vi "Agilent SNA Read Learn String.vi"(6 "Get SWP Learn String? (T)":bool=TRUE, 7 "Agilent SNA & SWP":T2, 8 "error in (no error)":errorcluster, 11 "VISA Resource Names":T1) -> (0 "error out":errorcluster, 1 "SWP Learn String":string, 2 "SNA Learn String":string, 3 "dup VISA Resource Names":T1)   [LabVIEW 2011]
uses:
  TypeDefs/Agilent SNA Instrument Info.ctl
  TypeDefs/Agilent SNA VISA.ctl
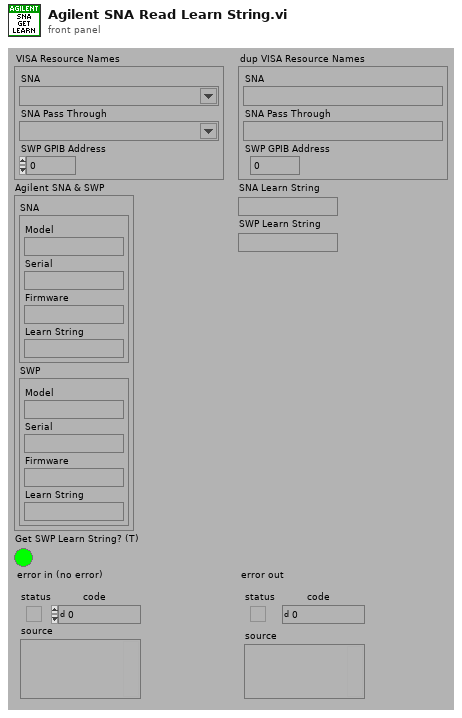
[diagram p1: front panel]
types:
  T1 = typedef "Agilent SNA VISA.ctl" = cluster{"SNA":refnum<visa-resource-name>, "SNA Pass Through":refnum<visa-resource-name>, "SWP GPIB Address":i32}
  T2 = typedef "Agilent SNA Instrument Info.ctl" = cluster{"SNA":cluster{"Model":string, "Serial":string, "Firmware":string, "Learn String":string}, "SWP":cluster{"Model":string, "Serial":string, "Firmware":string, "Learn String":string}}
  T3 = typedef "Agilent SNA Model.ctl" = enum16{"Not Supported", "8757X"}
  T4 = typedef "Agilent SNA SWP Model.ctl" = enum16{"Not Supported", "836XXX", "8375XX", "E82X7D"}
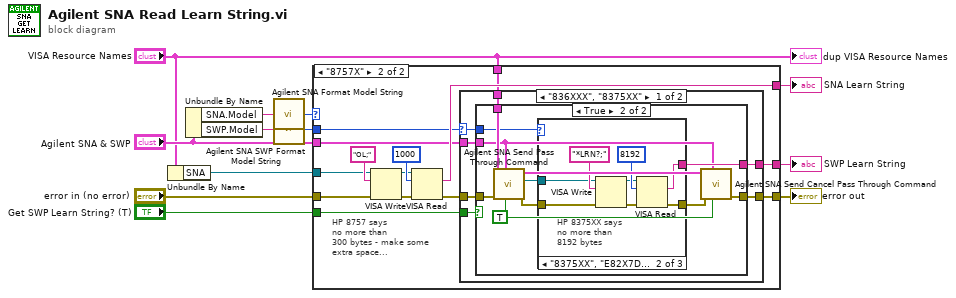
[diagram p0: block diagram]
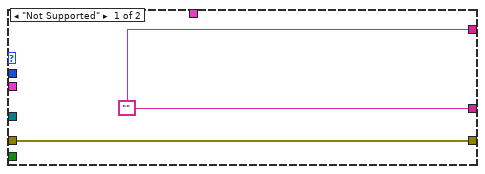
[diagram p2: hidden frame]
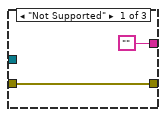
[diagram p4: hidden frame]
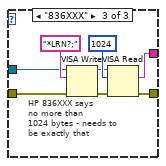
[diagram p5: hidden frame]
diagram:
  n1 = Unbundle By Name("VISA Resource Names") -> ("SNA"=w8:refnum<visa-resource-name>)
  n2 = Unbundle By Name("Agilent SNA & SWP") -> ("SNA.Model"=w9:string, "SWP.Model"=w3:string)
  n3 = call "Agilent SNA Format Model String.vi"("Model String"=w9) -> ("Model"=w10:T3)
  n4 = call "Agilent SNA SWP Format Model String.vi"("Model String"=w3) -> ("Model"=w2:T4)
  n5 = case shown="\"8757X\"" w10 {
    tunnel: w8 -> [_ w24]
    tunnel: [w13 w23] -> w12
    tunnel: "error in (no error)" -> [w14 w22]
    tunnel: [w14 w18] -> w7
    tunnel: [w13 w21] -> w6
    tunnel: "Agilent SNA & SWP" -> [_ w17]
    tunnel: "VISA Resource Names" -> [_ w19]
    tunnel: w2 -> [_ w15]
    tunnel: "Get SWP Learn String? (T)" -> [_ w16]
    frame "Not Supported" {
      w13 = ""
    }
    frame "8757X" {
      # "HP 8757 says\nno more than\n300 bytes - make some\nextra space..."
      n6 = VISA Write(VISA resource name=w24, write buffer="OL;", error in (no error)=w22) -> (VISA resource name out=w25:refnum<visa-resource-name>, error out=w27:errorcluster)  [unwired: 1 out]
      n7 = VISA Read(VISA resource name=w25, byte count=u32 1000, error in (no error)=w27) -> (read buffer=w23:string, error out=w20:errorcluster)  [unwired: 2 out]
      n8 = case shown="\"836XXX\", \"8375XX\"" w15 {
        selector: w15 -> [w29 _]
        tunnel: [w35 _] -> w21
        tunnel: w20 -> [w34 w66]
        tunnel: w19 -> [w33 _]
        tunnel: [w32 w66] -> w18
        tunnel: w17 -> [w31 _]
        tunnel: w16 -> [w30 _]
        frame "836XXX", "8375XX" {
          n9 = case shown="True" w30 {
            tunnel: [_ w45] -> w35
            tunnel: w34 -> [w36 w44]
            tunnel: w33 -> [_ w43]
            tunnel: [w36 w42] -> w32
            tunnel: w31 -> [_ w39]
            tunnel: w29 -> [_ w38]
            frame False {
            }
            frame True {
              w37 = TRUE ("SCPI? (F)")
              n10 = call "Agilent SNA Send Pass Through Command.vi"("SCPI? (F)"=w37, "Agilent SNA & SWP"=w39, "error in (no error)"=w44, "VISA Resource Names"=w43) -> ("error out"=w46:errorcluster, "SNA Pass Through"=w47:refnum<visa-resource-name>, "dup VISA Resource Names"=w40:T1)  [unwired: 5 out]
              n11 = case shown="\"8375XX\", \"E82X7D\"" w38 {
                tunnel: w47 -> [_ w53 w61]
                tunnel: ["" w52 w60] -> w45
                tunnel: w46 -> [w49 w51 w59]
                tunnel: [w49 w50 w58] -> w41
                frame "Not Supported" {
                }
                frame "8375XX", "E82X7D" {
                  # "HP 8375XX says\nno more than\n8192 bytes"
                  n12 = VISA Write(VISA resource name=w53, write buffer="*LRN?;", error in (no error)=w51) -> (VISA resource name out=w54:refnum<visa-resource-name>, error out=w56:errorcluster)  [unwired: 1 out]
                  n13 = VISA Read(VISA resource name=w54, byte count=u32 8192, error in (no error)=w56) -> (read buffer=w52:string, error out=w50:errorcluster)  [unwired: 2 out]
                }
                frame "836XXX" {
                  # "HP 836XXX says\nno more than\n1024 bytes - needs to\nbe exactly that"
                  n14 = VISA Write(VISA resource name=w61, write buffer="*LRN?;", error in (no error)=w59) -> (VISA resource name out=w62:refnum<visa-resource-name>, error out=w64:errorcluster)  [unwired: 1 out]
                  n15 = VISA Read(VISA resource name=w62, byte count=u32 1024, error in (no error)=w64) -> (read buffer=w60:string, error out=w58:errorcluster)  [unwired: 2 out]
                }
              }
              n16 = call "Agilent SNA Send Cancel Pass Through Command.vi"("SCPI? (F)"=w37, "Agilent SNA & SWP"=w39, "error in (no error)"=w41, "VISA Resource Names"=w40) -> ("error out"=w42:errorcluster)  [unwired: 7 out]
            }
          }
        }
        frame "Not Supported", "E82X7D" {
        }
      }
    }
  }
  "error out" <- w7
  "SNA Learn String" <- w12
  "SWP Learn String" <- w6
  "dup VISA Resource Names" <- "VISA Resource Names"
